vi "AlazarDSPGetNextBufferFloat.vi"(4 "error in (no error)":errorcluster, 5 "timeout_ms":u32, 6 "Buffer":sgl[](array[numeric]), 7 "Handle":u64) -> (0 "error out":errorcluster, 1 "Return Code":u32, 2 "Buffer":sgl[](array[numeric]), 3 "Handle":u64)   [LabVIEW 2018]
doc: "This function returns when the board has received sufficient trigger events to fill the buffer, or the timeout interval has elapsed. To use this function, AlazarBeforeAsyncRead must be called with the ADMA_ALLOC_BUFFERS flag."
uses:
  ATSApi.dll
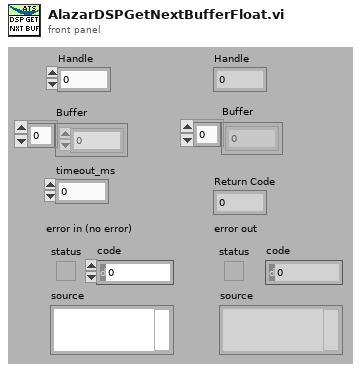
[diagram p1: front panel]
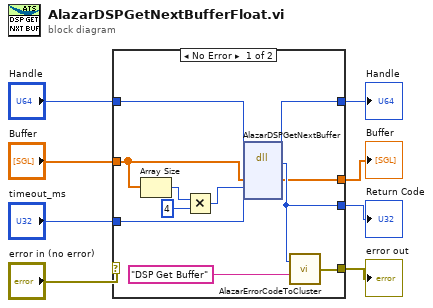
[diagram p0: block diagram]
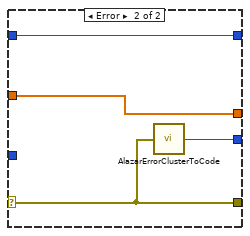
[diagram p2: hidden frame]
diagram:
  n1 = case shown="No Error" "error in (no error)" {
    selector: "error in (no error)" -> [_ w23]
    tunnel: [w16 w23] -> w7
    tunnel: [w18 w22] -> w6
    tunnel: "Handle" -> [w19 w21]
    tunnel: [w15 w21] -> w4
    tunnel: "Buffer" -> [w12 w20]
    tunnel: "timeout_ms" -> [w13 _]
    tunnel: [w14 w20] -> w1
    frame No Error {
      n2 = Array Size(array=w12) -> (size(s)=w10:i32)
      n3 = Multiply(x=w10, y=4) -> (x*y=w11:i32)
      n4 = dll-call lib="ATSApi.dll" fn="AlazarDSPGetNextBuffer"("handle"=w19, "buffer"=w12, "bytesToCopy"=w11, "timeout_ms"=w13) -> ("return type"=w18:u32, "handle"=w15:u64, "buffer"=w14:sgl[])  [unwired: 5 in, 2 out]
      n5 = call "AlazarErrorCodeToCluster.vi"("Message"="DSP Get Buffer", "Error Code"=w18) -> ("error out"=w16:errorcluster)
    }
    frame Error {
      n6 = call "AlazarErrorClusterToCode.vi"("error in (no error)"=w23) -> ("Error Code"=w22:u32)
    }
  }
  "Handle" <- w4
  "error out" <- w7
  "Return Code" <- w6
  "Buffer" <- w1
